vi "LiftExecute.vi"(8 "error in (no error)":errorcluster, 11 "Lift in":refnum<class "Lift.lvclass">) -> (0 "error out":errorcluster, 2 "Setpoint reached?":bool, 3 "Lift out":refnum<class "Lift.lvclass">)   [LabVIEW 2018, in "Lift.lvclass"]
uses:
  Lift.lvclass
  <vilib>/Rock Robotics/WPI/ThirdParty/Phoenix-LabVIEW/Motor Controller/Controls/CTRE_Phoenix_MotorControl_ControlMode.ctl
  Lift.lvclass/Lift.ctl
  9107f9ab-2796-41ff-83b2-5d61265c5f54.vi
  <vilib>/Rock Robotics/WPI/ThirdParty/Phoenix-LabVIEW/Motor Controller/Get/CTRE_Phoenix_MotorController_GetQuadratureData.vi
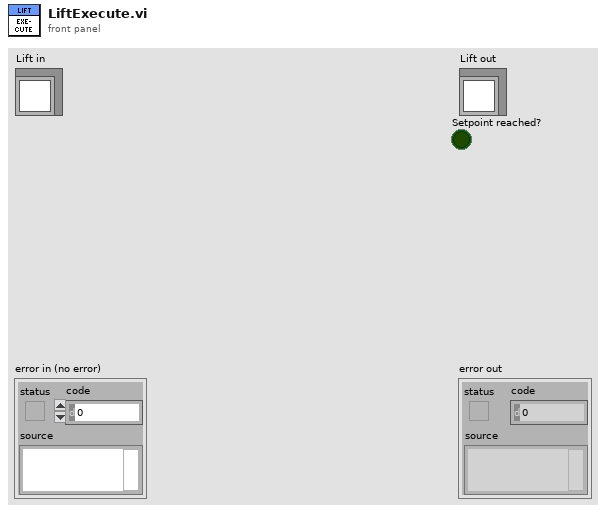
[diagram p1: front panel]
types:
  T1 = typedef "CTRE_Phoenix_MotorControl_ControlMode.ctl" = u16
  T2 = typedef "WPI_MotorControlDeviceRef.ctl" = cluster{"DeviceStatus":errorcluster, "Type":T3, "PWM":cluster{"PWM Channel":T4, "DeadBand":T5}, "CAN":cluster{"Device Number":u8, "SetOutput VI Ref":variant, "GetOutput VI Ref":variant, "Enable VI Ref":variant, "Disable VI Ref":variant, "Data":variant}, "Invert":bool, "DIO PWM":cluster{"PWM \"Enable\" Channel":T4, "DIOChannel":T6, "PWM Rate":dbl}}
  T3 = typedef "WPI_MotorControlType.ctl" = enum16{"PWM", "CAN", "DIO PWM"}
  T4 = typedef "FPGA_DIOPWMChannel.ctl" = enum8{"PWM 0", "PWM 1", "PWM 2", "PWM 3", "PWM 4", "PWM 5", "PWM 6", "PWM 7", "PWM 8", "PWM 9", "PWM MXP 0", "PWM MXP 1", "PWM MXP 2", "PWM MXP 3", "PWM MXP 4", "PWM MXP 5", "PWM MXP 6", "PWM MXP 7", "PWM MXP 8", "PWM MXP 9", "Invalid"}
  T5 = typedef "WPI_PWMDeadband.ctl" = cluster{"Name":string, "maxPositivePwm":i32, "minPositivePwm":i32, "centerPwm":i32, "maxNegativePwm":i32, "minNegativePwm":i32, "angularRange":u16}
  T6 = typedef "FPGA_DIOChannel.ctl" = enum8{"DIO 0", "DIO 1", "DIO 2", "DIO 3", "DIO 4", "DIO 5", "DIO 6", "DIO 7", "DIO 8", "DIO 9", "DIO MXP 0", "DIO MXP 1", "DIO MXP 2", "DIO MXP 3", "DIO MXP 4", "DIO MXP 5", "DIO MXP 6", "DIO MXP 7", "DIO MXP 8", "DIO MXP 9", "DIO MXP 10", "DIO MXP 11", "DIO MXP 12", "DIO MXP 13", "DIO MXP 14", "DIO MXP 15", "SPI Port CS1", "SPI Port CS2", "SPI Port CS3", "SPI Port MISO", "SPI Port MOSI", "Invalid"}
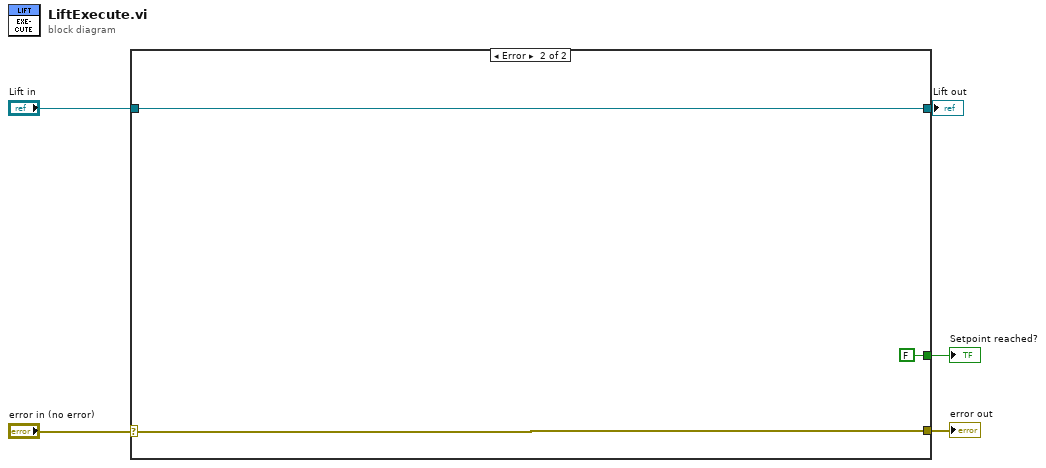
[diagram p0: block diagram]
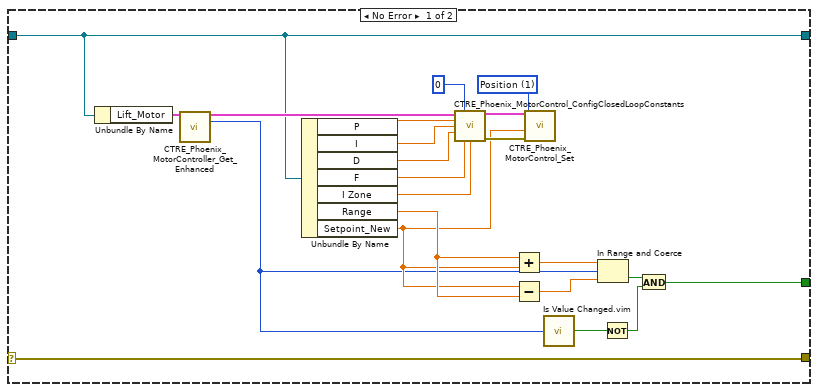
[diagram p2: hidden frame]
diagram:
  n1 = case shown="Error" "error in (no error)" {
    selector: "error in (no error)" -> [w27 w30]
    tunnel: [w27 w30] -> w4
    tunnel: [w6 w29] -> w2
    tunnel: "Lift in" -> [w6 w29]
    tunnel: [w7 FALSE] -> w1
    frame No Error {
      w16 = T1 1 items=["PercentOutput"=0, "Position"=1, "Velocity"=2, "Current"=3, "Follower"=5, "MotionProfile"=6, "MotionMagic"=7, "MotionProfileArc"=10, "Disabled"=15] ("Control Mode")
      n2 = Unbundle By Name(w6) -> ("Lift_Motor"=w26:T2)
      n3 = call-poly <vilib>:"CTRE_Phoenix_MotorController_Get_Enhanced.vi"("PhoenixMotorControlDevRef"=w26) -> ("PhoenixMotorControlDevRef"=w25:T2, "Quadrature Position"=w8:i32)  [unwired: 11 in, 2 out]
      n4 = Unbundle By Name(w6) -> ("P"=w24:dbl, "I"=w23:dbl, "D"=w22:dbl, "F"=w21:dbl, "I Zone"=w20:dbl, "Range"=w10:dbl, "Setpoint_New"=w9:dbl)
      n5 = call <vilib>:"CTRE_Phoenix_MotorControl_ConfigClosedLoopConstants.vi"("PhoenixMotorControlDevRef"=w25, "slotIdx"=0, "P"=w24, "I"=w23, "D"=w22, "F"=w21, "I Zone"=w20) -> ("PhoenixMotorControlDevRef"=w17:T2, "error out"=w18:errorcluster)  [unwired: 7 in]
      n6 = Add(x=w10, y=w9) -> (x+y=w14:dbl)
      n7 = Subtract(x=w9, y=w10) -> (x-y=w15:dbl)
      n8 = call <vilib>:"CTRE_Phoenix_MotorControl_Set.vi"("error in (no error)"=w18, "Output"=w9, "Control Mode"=w16, "PhoenixMotorControlDevRef"=w17) -> ()  [unwired: 6 in, 2 out]
      n9 = call "Is Value Changed.vim"("value"=w8) -> ("changed or first call?"=w11:bool)
      n10 = In Range and Coerce(upper limit=w14, x=w8, lower limit=w15) -> (In Range?=w13:bool)  [unwired: 1 out]
      n11 = Not(x=w11) -> (.not. x?=w12:bool)
      n12 = And(x=w13, y=w12) -> (x .and. y?=w7:bool)
    }
    frame Error {
    }
  }
  "error out" <- w4
  "Lift out" <- w2
  "Setpoint reached?" <- w1
